vi "Close.vi"(8 "error in":errorcluster, 11 "Cfg Dev in":refnum<class "Vaisala.lvclass">) -> (0 "error out":errorcluster, 3 "Cfg Dev out":refnum<class "Vaisala.lvclass">)   [LabVIEW 2015, in "Vaisala Library.lvlib" / "Vaisala.lvclass"]
uses:
  Vaisala.lvclass
  reusable/Session APIs/Serial/Serial Session.lvclass
  Vaisala.lvclass/Vaisala.ctl
  <vilib>/MSR Consulting, LLC/ESF/Session - Root.lvclass
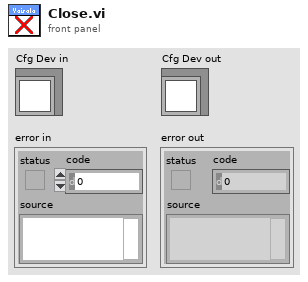
[diagram p1: front panel]
types:
  T1 = typedef "Session - Root.lvclass/Session Handle.ctl" = refnum<data-value>
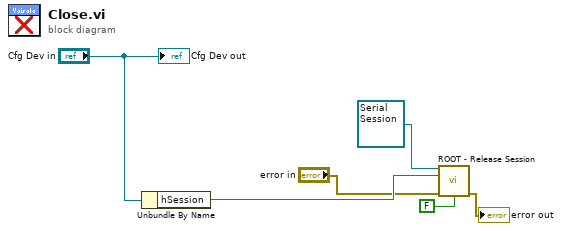
[diagram p0: block diagram]
diagram:
  n1 = Unbundle By Name("Cfg Dev in") -> ("hSession"=w5:T1)
  n2 = call <vilib>:"ROOT - Release Session.vi"("OBJ - Session in"=refnum<class "Serial Session.lvclass"> refnum ("Serial Session"), "Session Handle in"=w5, "error in (no error)"="error in", "force destroy? (F)"=FALSE) -> ("error out"=→"error out":errorcluster)  [unwired: 10 in, 1 out]
  "Cfg Dev out" <- "Cfg Dev in"
